vi "Configure AV Resistance Measurement.vi"(0 "VISA resource name":refnum<visa-resource-name>, 1 "Enable One Shot Mode (T: Enable)":bool=TRUE, 2 "AV Autoclear (T: Enable)":bool=TRUE, 5 "AV High Voltage (10 V)":dbl=10.0, 7 "AV Pulse Time (1 s)":dbl=1.0, 9 "AV Measurement Cycles (3)":i32=3, 11 "error in (no error)":errorcluster, 12 "AV Units (0: Amps)":u16(ring) items=["Amps", "Ohms"]) -> (4 "VISA resource name out":refnum<visa-resource-name>, 15 "error out":errorcluster)   [LabVIEW 2021, in "Keithley 648X Series.lvlib"]
doc: "Configures the AV (Alternating Voltage) Resistance Measurement function. The Alternating Voltage Resistance Measurement measures ohms by alternating between the configured high voltage output and a 0V output. This is especially useful when the resistance or device being measured exhibits high background or noise currents. AV results are stored in the data buffer.\n\n<b>Notes:</b>\n1)In order to arm the AV Resistance Measurement function you must use the <b>Arm AV Measurement</b> action VI.\n2)<b>This VI supports Model 6487 only</b>"
uses:
  <instrlib>/Keithley 648X Series/Keithley 648X Series.lvlib
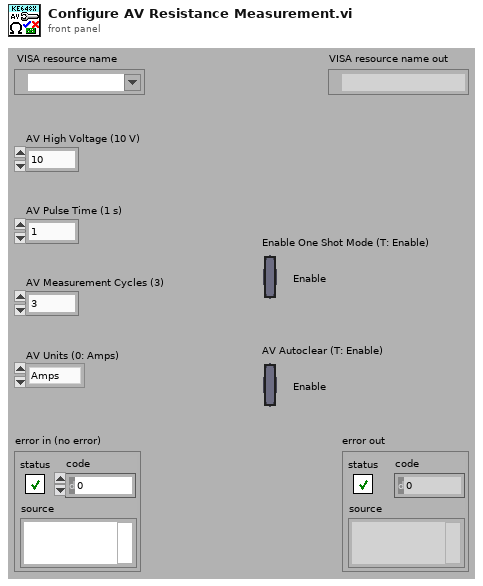
[diagram p1: front panel]
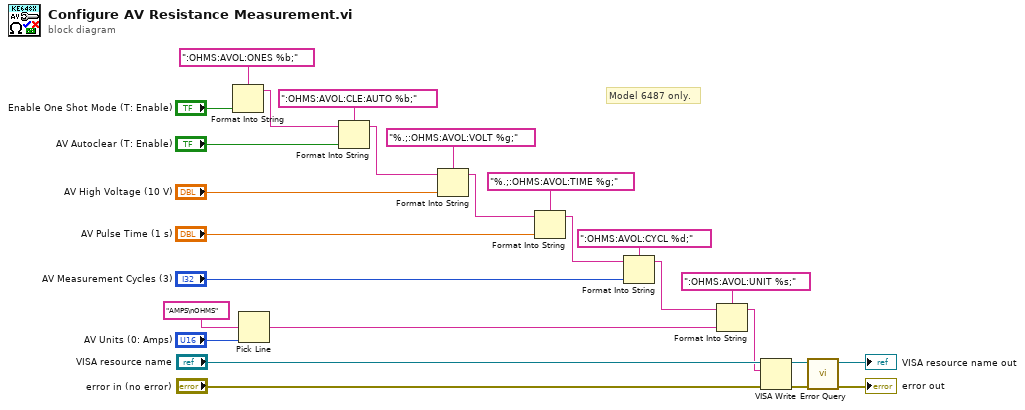
[diagram p0: block diagram]
diagram:
  # "Model 6487 only."
  n1 = Format Into String(format string=":OHMS:AVOL:ONES %b;", "Enable One Shot Mode (T: Enable)") -> (resulting string=w17:string)  [unwired: 2 in, 1 out]
  n2 = Pick Line(multi-line string="AMPS\nOHMS", line index="AV Units (0: Amps)") -> (output string=w2:string)  [unwired: 1 in]
  n3 = Format Into String(format string=":OHMS:AVOL:CLE:AUTO %b;", initial string=w17, "AV Autoclear (T: Enable)") -> (resulting string=w14:string)  [unwired: 1 in, 1 out]
  n4 = Format Into String(format string="%.;:OHMS:AVOL:VOLT %g;", initial string=w14, "AV High Voltage (10 V)") -> (resulting string=w11:string)  [unwired: 1 in, 1 out]
  n5 = Format Into String(format string="%.;:OHMS:AVOL:TIME %g;", initial string=w11, "AV Pulse Time (1 s)") -> (resulting string=w8:string)  [unwired: 1 in, 1 out]
  n6 = Format Into String(format string=":OHMS:AVOL:CYCL %d;", initial string=w8, "AV Measurement Cycles (3)") -> (resulting string=w5:string)  [unwired: 1 in, 1 out]
  n7 = Format Into String(format string=":OHMS:AVOL:UNIT %s;", initial string=w5, w2) -> (resulting string=w1:string)  [unwired: 1 in, 1 out]
  n8 = VISA Write(VISA resource name="VISA resource name", write buffer=w1, error in (no error)="error in (no error)") -> (VISA resource name out=w22:refnum<visa-resource-name>, error out=w21:errorcluster)  [unwired: 1 out]
  n9 = call <instrlib>:"Error Query.vi"("error in (no error)"=w21, "VISA resource name"=w22) -> ("error out"=→"error out":errorcluster, "VISA resource name out"=→"VISA resource name out":refnum<visa-resource-name>)  [unwired: 6 in, 2 out]
